vi "get echarts JS.vi"(8 "error in (no error)":errorcluster caption="错误输入（无错误）") -> (0 "error out":errorcluster)   [LabVIEW 2016, in "数据查询.lvlib"]
uses:
  <vilib>/httpClient/LabVIEWHTTPClient.lvlib
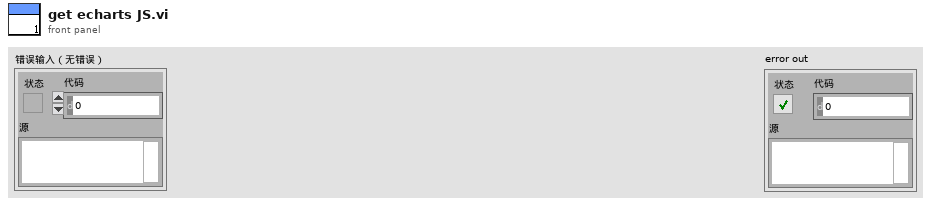
[diagram p1: front panel]
types:
  T1 = typedef "LabVIEWHTTPClient.lvlib/ClientHandle.ctl" = refnum<k1>
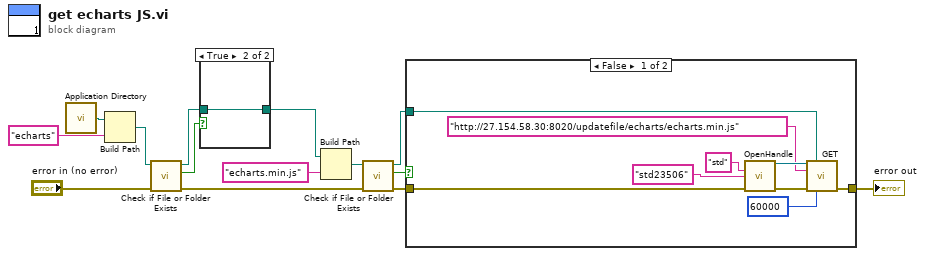
[diagram p0: block diagram]
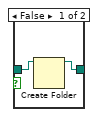
[diagram p3: hidden frame]
diagram:
  n1 = call <vilib>:"Application Directory.vi"() -> ("Application Directory"=w14:path)
  n2 = Build Path(base path=w14, name or relative path="echarts" ("名称或相对路径")) -> (appended path=w12:path)
  n3 = call <vilib>:"Check if File or Folder Exists.vi"("error in (no error)"="error in (no error)", "path"=w12) -> ("error out"=w3:errorcluster, "file or folder exists?"=w11:bool, "dup path"=w10:path)  [unwired: 7 in]
  n4 = case shown="True" w11 {
    tunnel: w10 -> [w16 w17]
    tunnel: [w15 w17] -> w9
    frame False {
      n5 = Create Folder(path (use dialog)=w16) -> (created path=w15:path)  [unwired: 2 in, 2 out]
    }
    frame True {
    }
  }
  n6 = Build Path(base path=w9, name or relative path="echarts.min.js" ("名称或相对路径")) -> (appended path=w7:path)
  n7 = call <vilib>:"Check if File or Folder Exists.vi"("error in (no error)"=w3, "path"=w7) -> ("error out"=w4:errorcluster, "file or folder exists?"=w5:bool, "dup path"=w6:path)  [unwired: 7 in]
  n8 = case shown="False" w5 {
    tunnel: w6 -> [w21 _]
    tunnel: [w20 w27] -> w2
    tunnel: w4 -> [w19 w27]
    frame False {
      n9 = call <vilib>:"OpenHandle.vi"("username"="std", "password"="std23506", "error in (no error)"=w19) -> ("client handle out"=w25:T1, "error out"=w26:errorcluster)  [unwired: 11 in]
      n10 = call <vilib>:"GET.vi"("client handle"=w25, "output file"=w21, "url"="http://27.154.58.30:8020/updatefile/echarts/echarts.min.js" ("remote path"), "error in (no error)"=w26, "timeout (10000)"=60000) -> ("error out"=w20:errorcluster)  [unwired: 7 in, 3 out]
    }
    frame True {
    }
  }
  "error out" <- w2
